vi "Main(1).vi"() -> ()   [LabVIEW 2020]
doc: "Use this template to build a simple state machine design pattern. Each state executes code and determines which state to transition to."
uses:
  controls/State.ctl
  controls/Data.ctl
  <vilib>/daqmxs/DAQmx sim.lvlib
  <vilib>/Utility/TDMS File Viewer/NI_TDMS File Viewer.lvlib
  <vilib>/daqmxs/DAQmx Read sim (Analog Wfm 1Chan NSamp).vi
  <vilib>/DAQmx/configure/timing.llb/DAQmx Timing (Sample Clock).vi
  <vilib>/DAQmx/create/channels.llb/DAQmx Create Channel (AI-Voltage-Basic).vi
panel:
  out "Array":dbl[](array[numeric])
  out "x = y?":bool
  in  "Vyhledat cislo":bool
  in  "Numeric":dbl
  in  "file in":path
  in  "Zobrazit zmerena data":bool
  out "Waveform Graph":waveform(dbl)(graph)
  in  "physical channels":tag
  in  "Do Something Else <Replace Me>":bool
  in  "Zmerit data":bool
  in  "Exit":bool
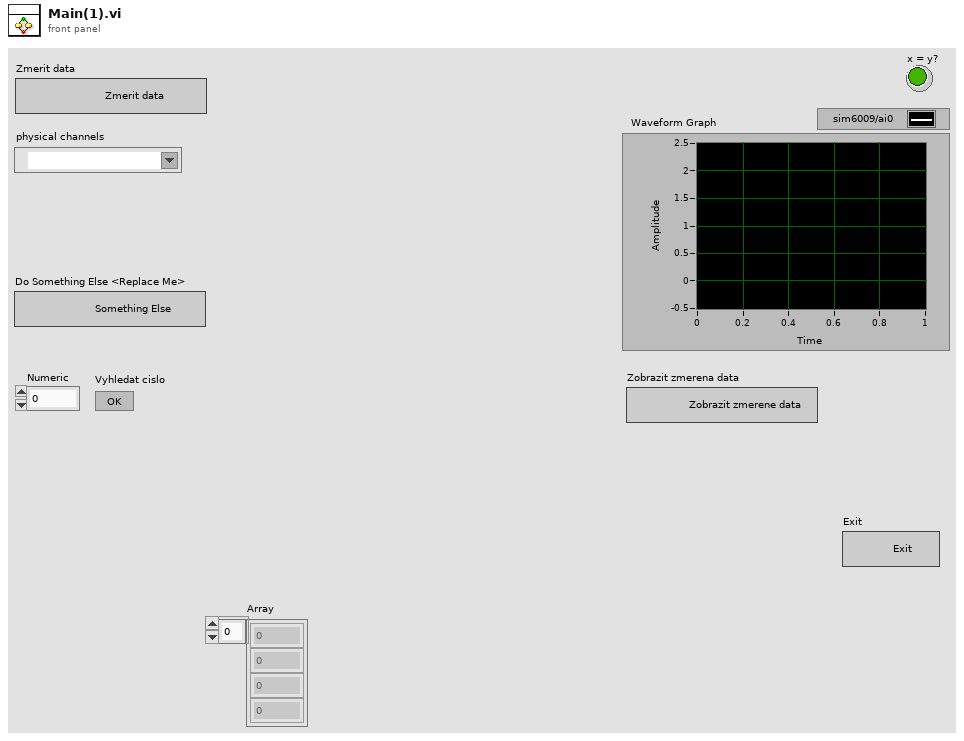
[diagram p1: front panel]
types:
  T1 = typedef "Data.ctl" = cluster{"Boolean <Replace Me>":bool, "String <Replace Me>":string, "Numeric <Replace Me>":dbl}
  T2 = typedef "State.ctl" = enum16{"Initialize", "Wait for Event", "User State 1", "User State 2", "Exit"}
  T3 = enum16{"open", "open or create", "create or replace", "create", "open (read-only)"}
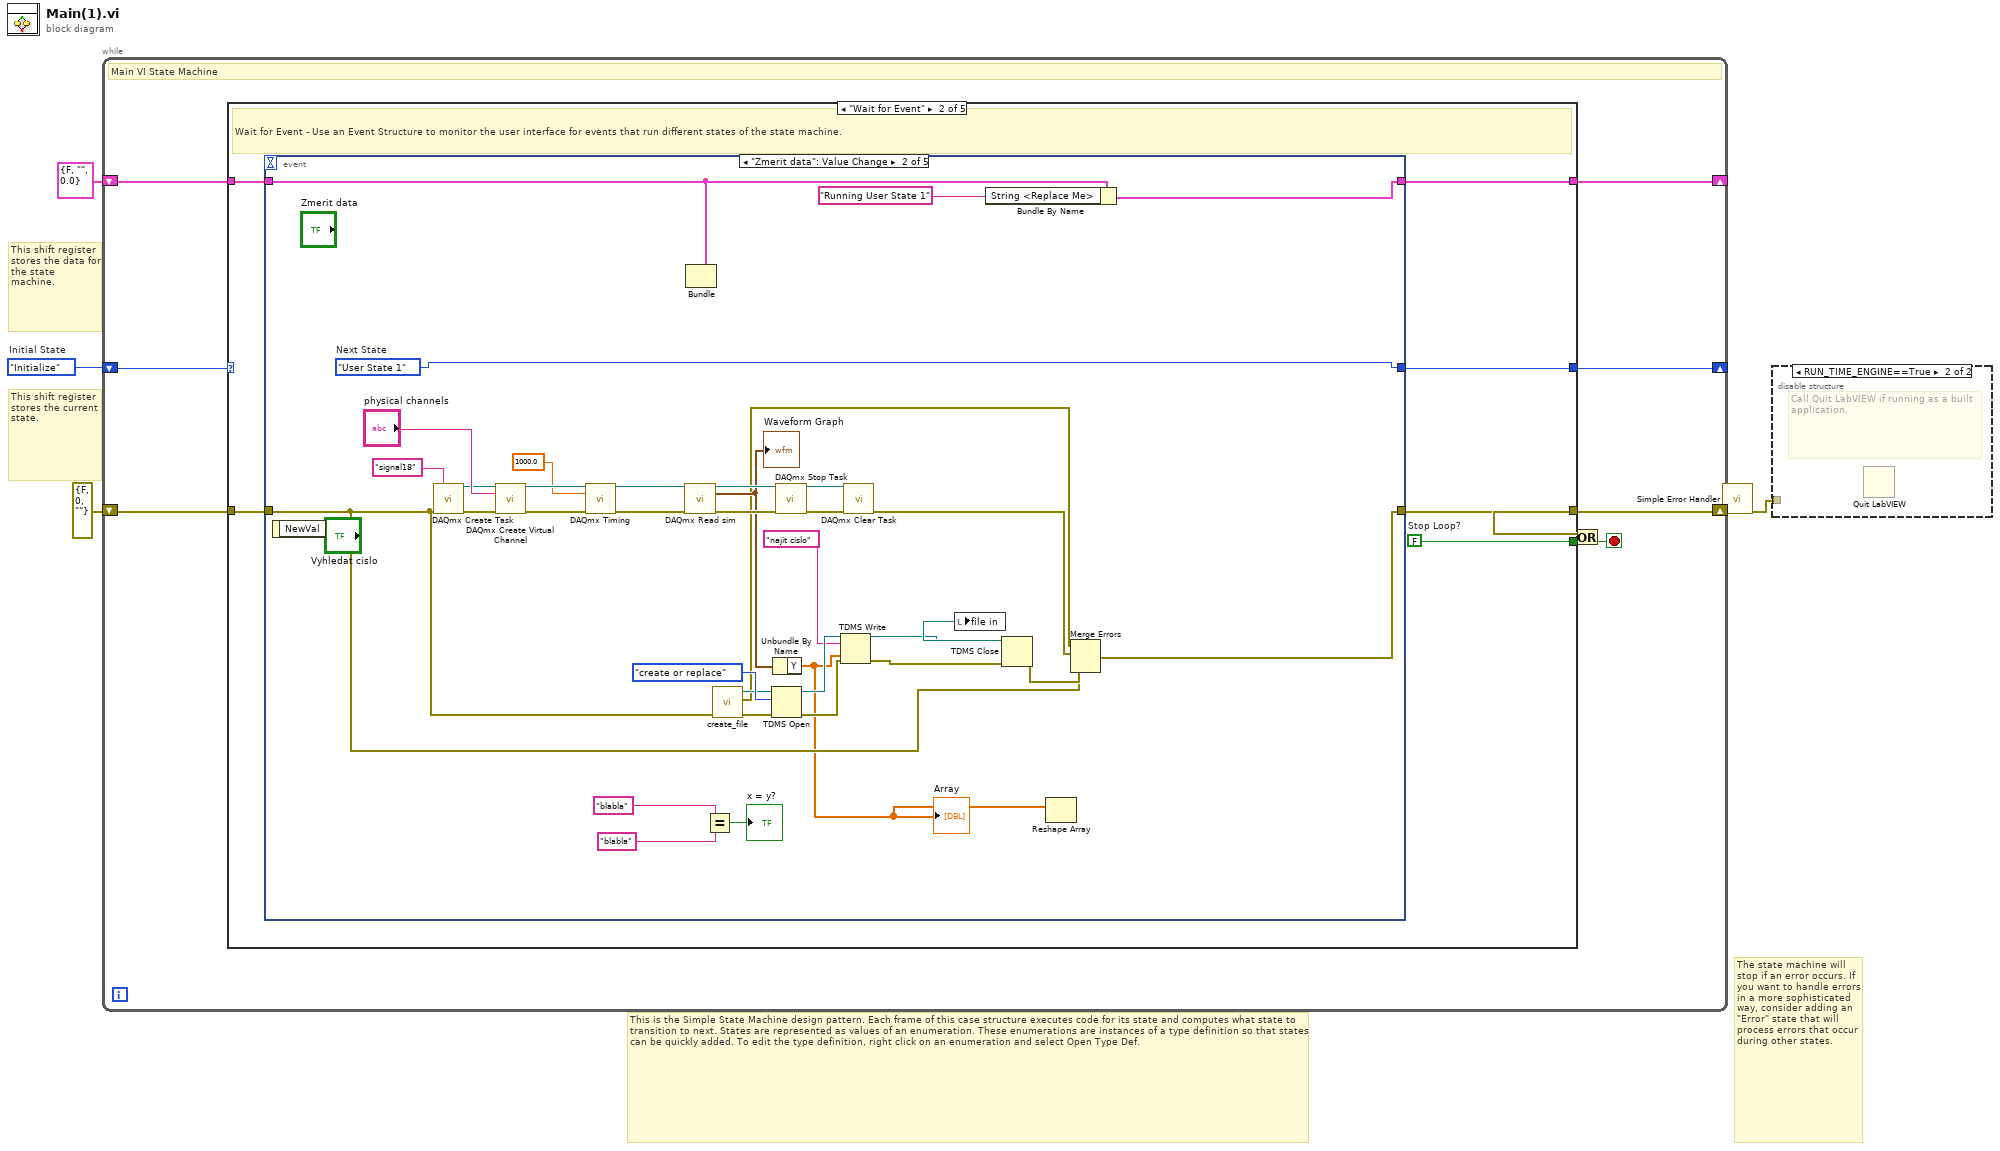
[diagram p0: block diagram]
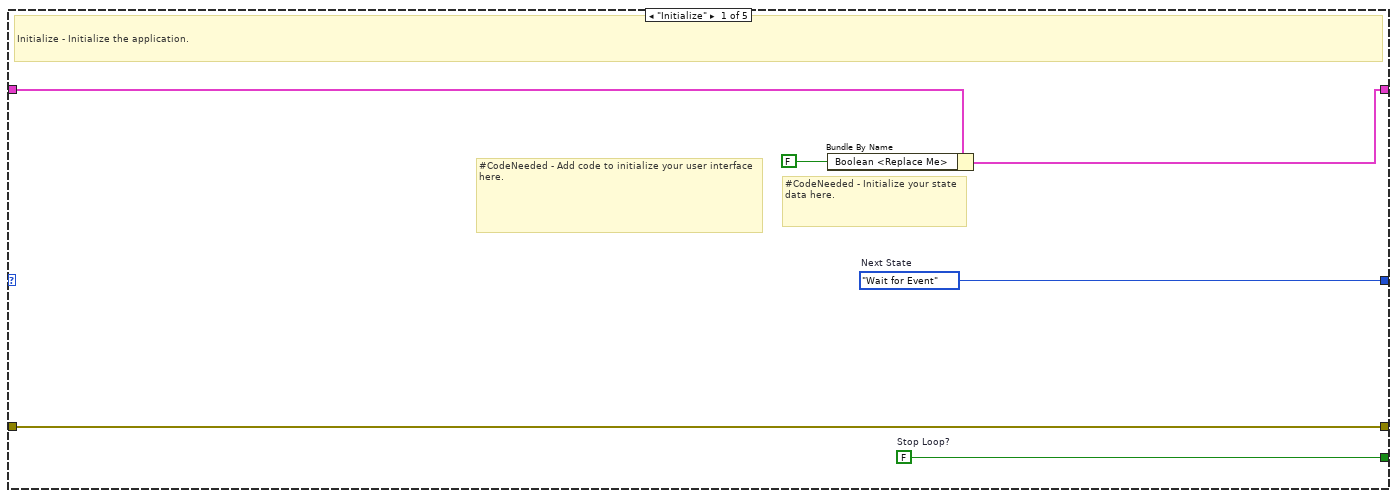
[diagram p3: hidden frame]
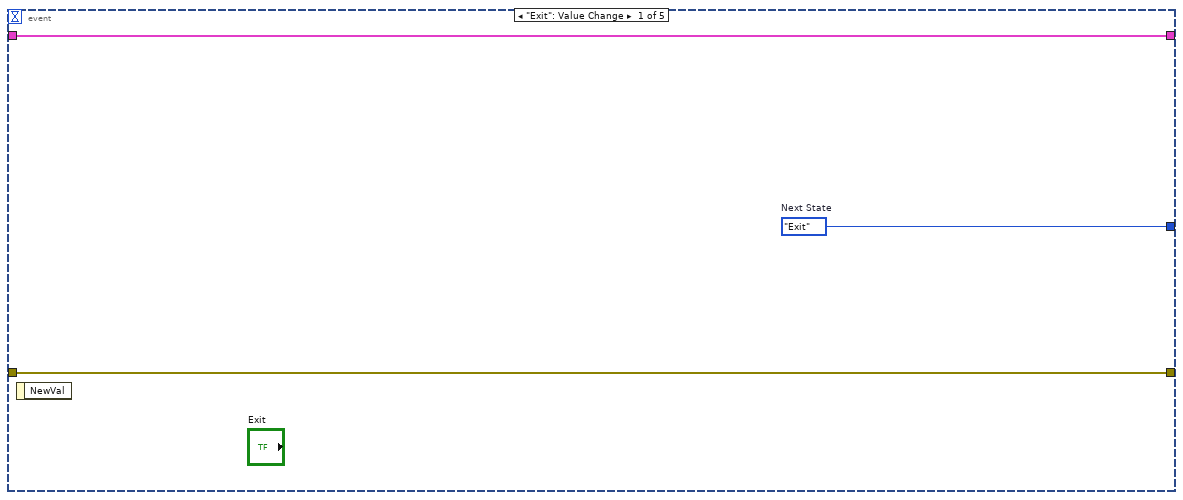
[diagram p4: hidden frame]
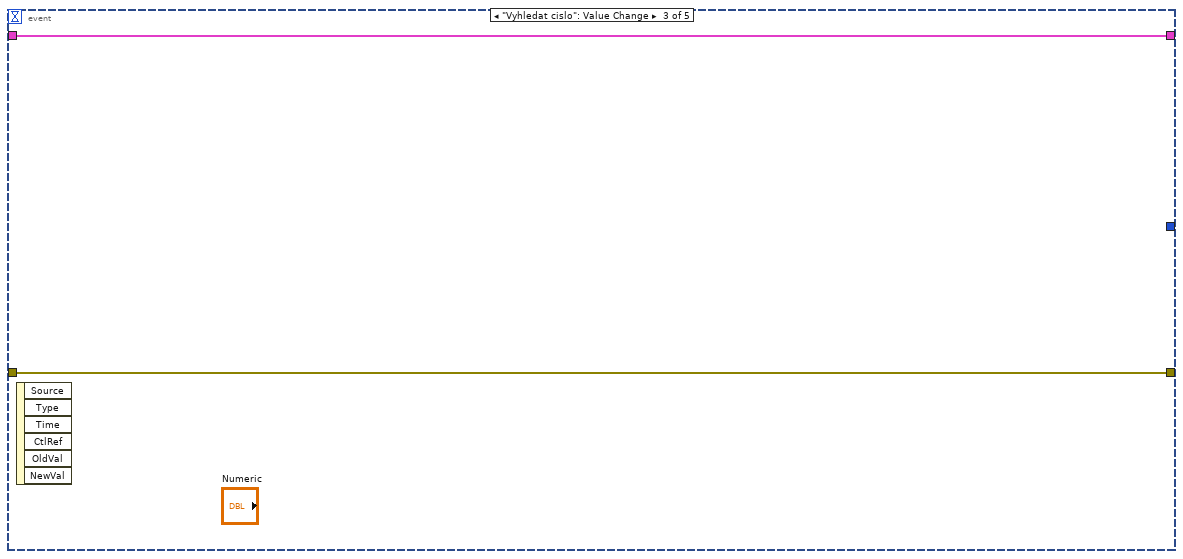
[diagram p5: hidden frame]
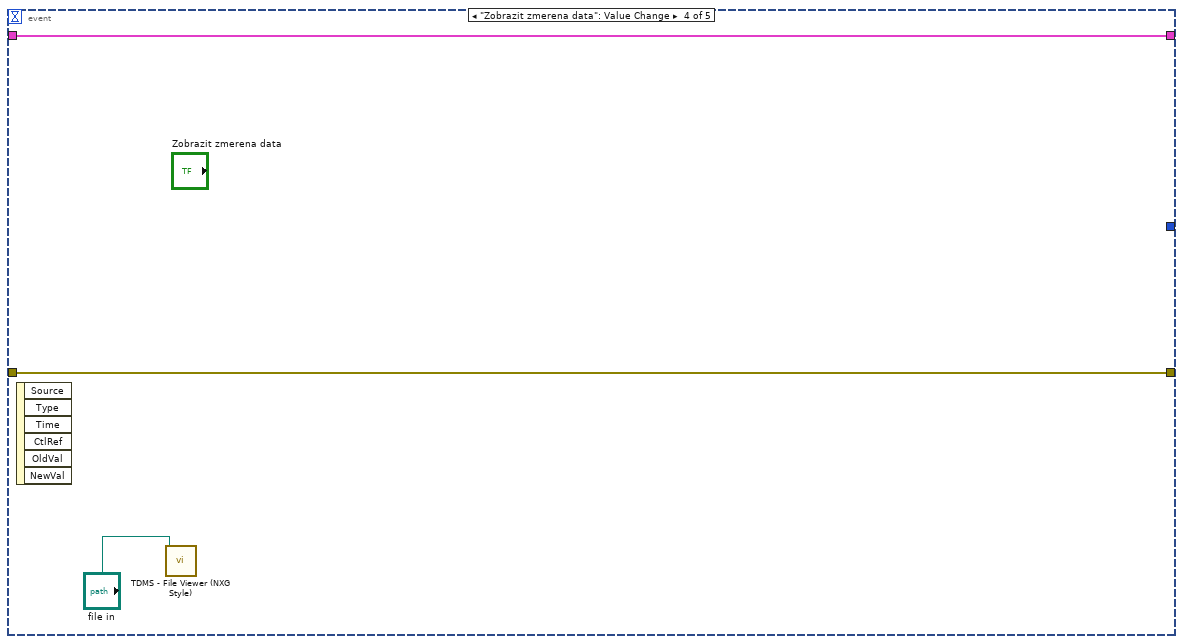
[diagram p6: hidden frame]
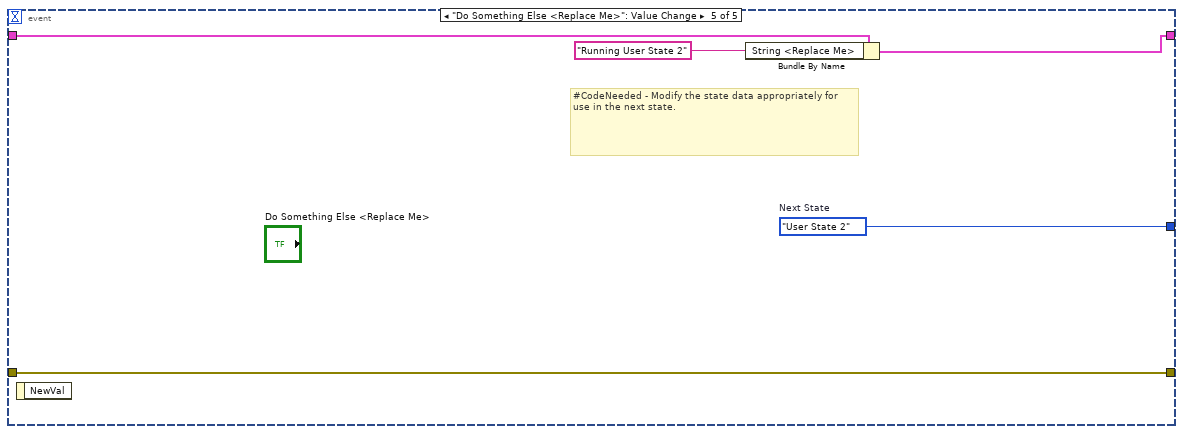
[diagram p7: hidden frame]
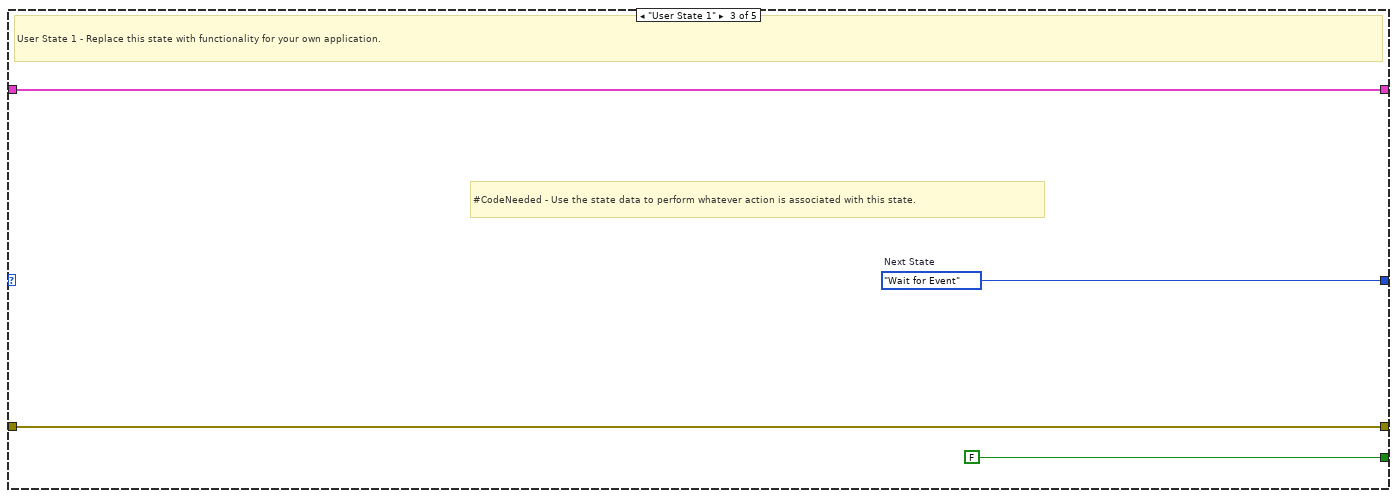
[diagram p8: hidden frame]
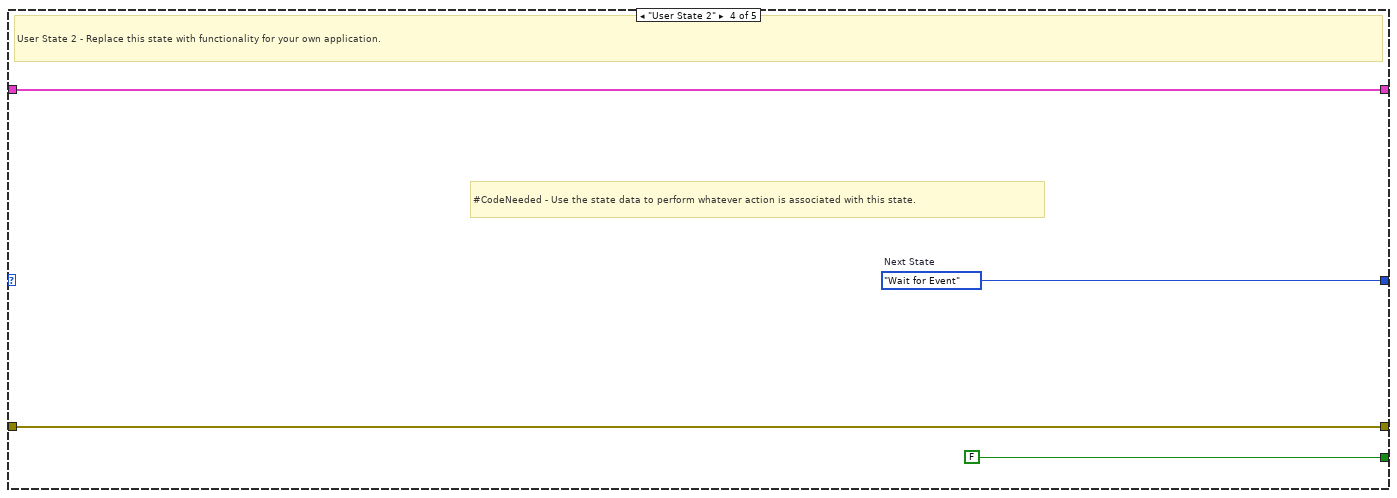
[diagram p9: hidden frame]
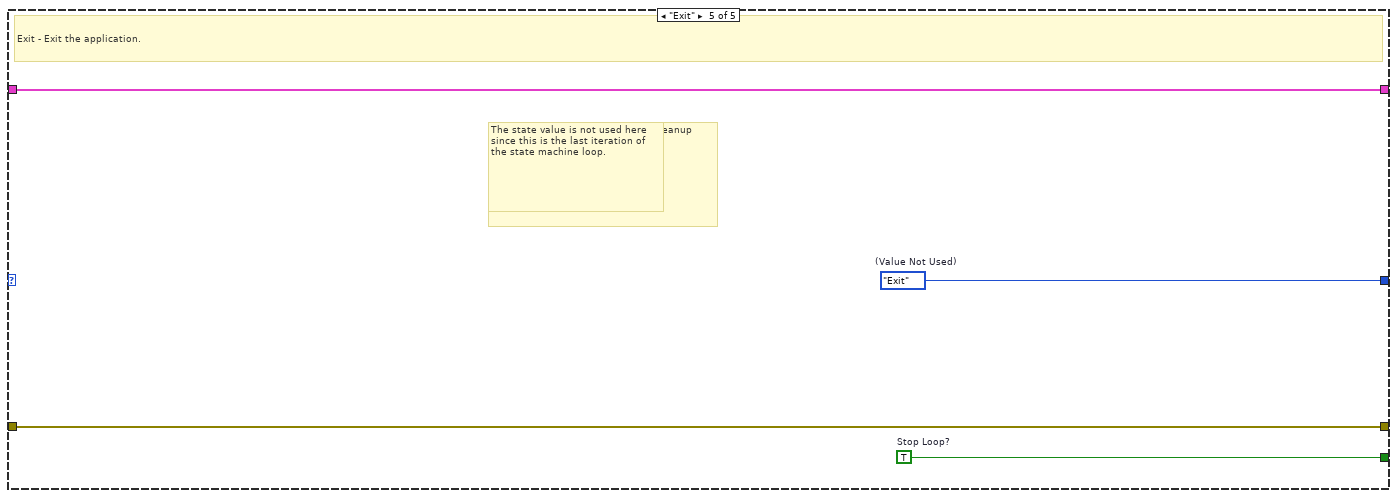
[diagram p10: hidden frame]
diagram:
  w5 = State."Initialize"  # Initial State
  # "The state machine will stop if an error occurs. If you want to handle errors in a more sophisticated way, consider adding an \"Error\" state that will process errors that occur during other states."
  # "This shift register stores the data for the state machine."
  # "This is the Simple State Machine design pattern. Each frame of this case structure executes code for its state and computes what state to transition to next. States are represented as values of an enumeration. These enumerations are instances of a type definition so that states can be quickly added. To edit the type definition, right click on an enumeration and select Open Type Def."
  # "This shift register stores the current state."
  n1 = while {
    shift-right: [w12] -> _
    shift-left: w5 -> [w13]
    shift-right: [w10] -> _
    shift-left: T1 {"Boolean <Replace Me>"=FALSE, "String <Replace Me>"="", "Numeric <Replace Me>"=0.0} ("Data") -> [w11]
    shift-right: [w6] -> w2
    shift-left: errorcluster {"status"=FALSE, "code"=0, "source"=""} ("error constant") -> [w9]
    stop <- w7 stop-if-true
    # "Main VI State Machine"
    n2 = case shown="\"Wait for Event\"" w13 {
      tunnel: [w19 w25 w78 w82 w86] -> w12
      tunnel: [w18 w24 FALSE ("Stop Loop?") FALSE ("Stop Loop?") w84] -> w8
      tunnel: w11 -> [w17 w23 w76 w80 w85]
      tunnel: [w16 w22 w76 w80 w85] -> w10
      tunnel: w9 -> [w14 w21 w75 w79 w83]
      tunnel: [w14 w20 w75 w79 w83] -> w6
      frame "Initialize" {
        w18 = FALSE  # Stop Loop?
        w19 = State."Wait for Event"  # Next State
        # "#CodeNeeded - Initialize your state data here."
        # "#CodeNeeded - Add code to initialize your user interface here."
        # "Initialize - Initialize the application."
        n3 = Bundle By Name(cluster=w17, "Boolean <Replace Me>"=FALSE ("Replace_Me_Boolean")) -> (w16:T1)
      }
      frame "Wait for Event" {
        w24 = FALSE  # Stop Loop?
        # "Wait for Event - Use an Event Structure to monitor the user interface for events that run different states of the state machine."
        n4 = event shown="[1] \"Zmerit data\": Value Change" {
          selector: _ -> [_ _ _ _ _]
          dyn-events: _ -> [_ _ _ _ _]
          timeout: _ -> [_ _ _ _ _]
          tunnel: [w28 w64 _ _ w74] -> w25
          tunnel: w23 -> [w27 w48 w66 w69 w73]
          tunnel: [w27 w63 w66 w69 w72] -> w22
          tunnel: w21 -> [w26 w37 w65 w68 w70]
          tunnel: [w26 w38 w65 w68 w70] -> w20
          event "Exit": Value Change {
            w28 = State."Exit"  # Next State
            n5 = event-data() -> ()  [unwired: 1 in, 1 out]
          }
          event "Zmerit data": Value Change {
            w64 = State."User State 1"  # Next State
            n6 = event-data() -> ()  [unwired: 1 in, 1 out]
            n7 = call <vilib>:"DAQmx Create Task.vi"("new task name"="signal18", "error in"=w37) -> ("task out"=w51:refnum<k21>, "error out"=w52:errorcluster)  [unwired: 12 in]
            n8 = call-poly <vilib>:"DAQmx Create Virtual Channel.vi"("task in"=w51, "physical channels"="physical channels", "error in"=w52) -> ("task out"=w54:refnum<k21>, "error out"=w55:errorcluster)  [unwired: 11 in]
            n9 = call-poly <vilib>:"DAQmx Timing.vi"("task/channels in"=w54, "rate"=1000.0, "error in"=w55) -> ("task out"=w56:refnum<k21>, "error out"=w57:errorcluster)  [unwired: 11 in]
            n10 = call-poly <vilib>:"DAQmx Read sim.vi"("task/channels in"=w56, "error in"=w57) -> ("task out"=w58:refnum<k21>, "data"=w47:waveform(dbl), "error out"=w59:errorcluster)  [unwired: 11 in]
            "Waveform Graph" <- w47
            n11 = Bundle(cluster=w48) -> ()  [unwired: 3 in, 1 out]
            n12 = Equal?(x="blabla", y="blabla") -> (x = y?=→"x = y?":bool)
            n13 = call "create_file.vi"("error in (no error)"=w37) -> (0:"error out"=w40:errorcluster, 2:"error out"=w35:errorcluster, "appended path"=w43:path)  [unwired: 8 in]
            n14 = TDMS Open(8:w40, 10:T3."create or replace" ("operation (0:open)"), 11:w43) -> (0:w42:errorcluster, 3:w45:refnum<k34>)  [unwired: 4 in]
            n15 = Unbundle By Name(w47) -> ("Y"=w29:dbl[])
            "Array" <- w29
            n16 = call <vilib>:"DAQmx Stop Task.vi"("task/channels in"=w58, "error in"=w59) -> ("task out"=w60:refnum<k21>, "error out"=w61:errorcluster)  [unwired: 12 in]
            n17 = TDMS Write(0:w45, 5:"najit cislo" ("group name in (Untitled)"), 9:w29, 11:w42) -> (4:w33:refnum<k34>, 15:w41:errorcluster)  [unwired: 2 in, 2 out]
            n18 = call <vilib>:"DAQmx Clear Task.vi"("task in"=w60, "error in"=w61) -> ("error out"=w36:errorcluster)  [unwired: 13 in]
            n19 = Bundle By Name(cluster=w48, "String <Replace Me>"="Running User State 1" ("Running User State 1")) -> (w63:T1)
            n20 = TDMS Close(8:w41, 11:w33) -> (0:w39:errorcluster, 3:w34:path)
            n21 = local write "file in"(w34) -> ()
            n22 = Reshape Array(w29) -> ()  [unwired: 1 in, 1 out]
            n23 = Merge Errors(w35, w36, w39, w37) -> (w38:errorcluster)
          }
          event "Vyhledat cislo": Value Change {
            n24 = event-data() -> ()  [unwired: 1 in, 6 out]
          }
          event "Zobrazit zmerena data": Value Change {
            n25 = event-data() -> ()  [unwired: 1 in, 6 out]
            n26 = call <vilib>:"TDMS - File Viewer (NXG Style).vi"("file in"="file in") -> ()  [unwired: 9 in, 2 out]
          }
          event "Do Something Else <Replace Me>": Value Change {
            w74 = State."User State 2"  # Next State
            # "#CodeNeeded - Modify the state data appropriately for use in the next state."
            n27 = event-data() -> ()  [unwired: 1 in, 1 out]
            n28 = Bundle By Name(cluster=w73, "String <Replace Me>"="Running User State 2" ("Running User State 2")) -> (w72:T1)
          }
        }
      }
      frame "User State 1" {
        w78 = State."Wait for Event"  # Next State
        # "#CodeNeeded - Use the state data to perform whatever action is associated with this state."
        # "User State 1 - Replace this state with functionality for your own application."
      }
      frame "User State 2" {
        w82 = State."Wait for Event"  # Next State
        # "#CodeNeeded - Use the state data to perform whatever action is associated with this state."
        # "User State 2 - Replace this state with functionality for your own application."
      }
      frame "Exit" {
        w84 = TRUE  # Stop Loop?
        w86 = State."Exit"  # (Value Not Used)
        # "#CodeNeeded - Add any required cleanup code here."
        # "The state value is not used here since this is the last iteration of the state machine loop."
        # "Exit - Exit the application."
      }
    }
    n29 = Or(x=w6, y=w8) -> (x .or. y?=w7:bool)
  }
  n30 = call <vilib>:"Simple Error Handler.vi"("error in (no error)"=w2) -> ("error out"=w1:errorcluster)  [unwired: 4 in, 4 out]
  n31 = disable-structure shown="RUN_TIME_ENGINE==True" {
    disable-tunnel: w1 -> [_ _]
    frame condition #0 (active) {
    }
    frame condition #1 {
      # "Call Quit LabVIEW if running as a built application."
      n32 = Quit LabVIEW() -> ()  [unwired: 1 in]
    }
  }
